vi "SMO.Example.ListStaticDependencies.vi"(8 "error in (no error)":errorcluster, 11 "SMO.Example":refnum<class "SMO.TopLevel.lvclass">) -> (0 "error out":errorcluster, 2 "Dependency Names":string[](array[string]), 3 "SMO.Example out":refnum<class "SMO.TopLevel.lvclass">)   [LabVIEW 2021, in "SMO.TopLevel.lvclass"]
doc: "---------------------------------------------------------------\nJKI State Machine Objects™\nhttp://jki.net/state-machine-objects/\nCopyright (C) 2005-2015, JKI <info@jki.net>\nALL RIGHTS RESERVED"
uses:
  SMO.TopLevel.lvclass
  C:/Repositories/SMO/src/SMO/SMO.lvclass
  src/SMO/SMO.lvclass
panel:
  # "For instructions on how to use the JKI State Machine Objects, examples and video tutorials, visit:\nhttp://jki.net/state-machine-objects/\n\nJKI State Machine Objects™\nhttp://jki.net/state-machine-objects/\nCopyright (C) 2005-2015, JKI <info@jki.net>\nALL RIGHTS RESERVED"
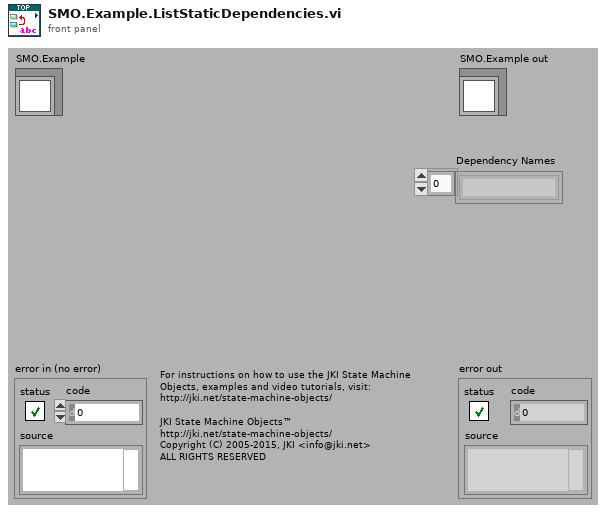
[diagram p1: front panel]
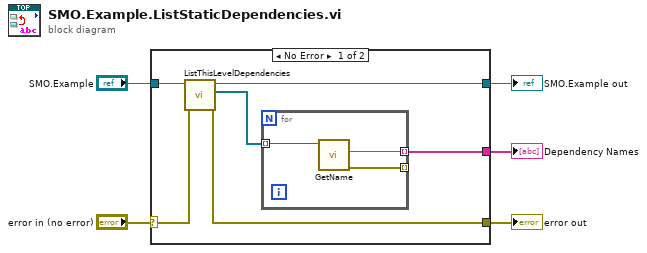
[diagram p0: block diagram]
diagram:
  n1 = case shown="No Error" "error in (no error)" {
    selector: "error in (no error)" -> [w6 w15]
    tunnel: "SMO.Example" -> [w7 w16]
    tunnel: [w10 w15] -> w4
    tunnel: [w11 w16] -> w3
    tunnel: [w9 _] -> w1
    frame No Error {
      n2 = call "ListThisLevelDependencies.vi"("error in (no error)"=w6, "SMO in"=w7) -> ("error out"=w10:errorcluster, "[My Dependencies]"=w8:refnum<class "SMO.lvclass">[], "SMO out"=w11:refnum<class "SMO.TopLevel.lvclass">)  [unwired: 7 in]
      n3 = for {
        tunnel: w8 -> [w14] mode=indexing
        tunnel: [w13] -> w9 mode=indexing
        tunnel: [w12] -> _ mode=indexing
        n4 = call "GetName.vi"("SMO"=w14) -> ("error out"=w12:errorcluster, "Name"=w13:string)  [unwired: 7 in, 2 out]
      }
    }
    frame Error {
    }
  }
  "error out" <- w4
  "SMO.Example out" <- w3
  "Dependency Names" <- w1
